vi "Service.EnumToGUID.vi"(11 "Type":T1) -> (3 "GUID":string)   [LabVIEW 2019, in "Diagnostics Addon System Explorer.lvlib"]
uses:
  Diagnostics Addon System Explorer.lvlib
  Addon Shared/SubVIs/Constants.vi
  Addon Shared/Diagnostics Addon Shared.lvlib
  Addon Shared/Types/Type.ctl
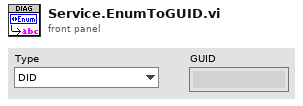
[diagram p1: front panel]
types:
  T1 = typedef "Diagnostics Addon Shared.lvlib/Type.ctl" = enum16{"DID", "CDID", "PID", "CPID", "Read Memory", "Write Memory", "IO Control", "Routine Start", "Routine Request", "Routine Stop", "User Defined", "DTC Control", "Clear DTCs", "Read DTCs", "Start DTCs", "DTC Change Count", "Tester Present", "Unlock ECU", "Reset ECU", "Diag Session Control", "Communication Control", "DPID Control", "Poll Control", "Diag Comm Port Control"}
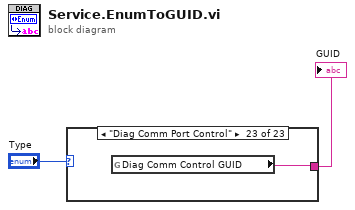
[diagram p0: block diagram]
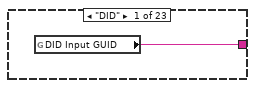
[diagram p2: hidden frame]
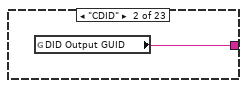
[diagram p3: hidden frame]
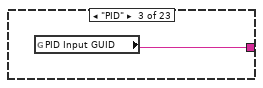
[diagram p4: hidden frame]
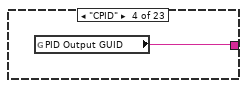
[diagram p5: hidden frame]
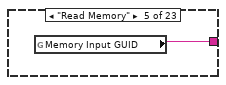
[diagram p6: hidden frame]
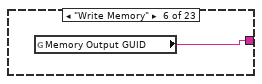
[diagram p7: hidden frame]
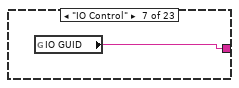
[diagram p8: hidden frame]
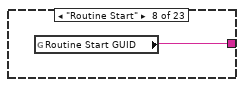
[diagram p9: hidden frame]
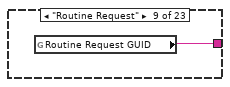
[diagram p10: hidden frame]
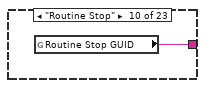
[diagram p11: hidden frame]
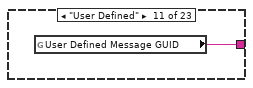
[diagram p12: hidden frame]
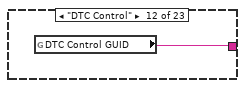
[diagram p13: hidden frame]
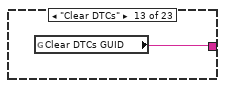
[diagram p14: hidden frame]
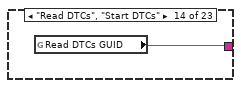
[diagram p15: hidden frame]
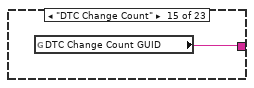
[diagram p16: hidden frame]
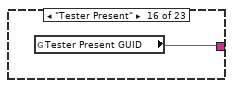
[diagram p17: hidden frame]
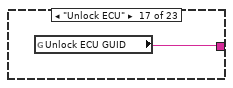
[diagram p18: hidden frame]
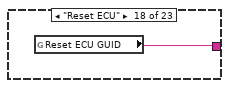
[diagram p19: hidden frame]
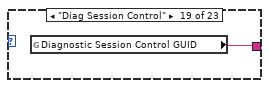
[diagram p20: hidden frame]
diagram:
  n1 = case shown="\"Diag Comm Port Control\"" "Type" {
    tunnel: [w3 w4 w5 w6 w7 w8 w9 w10 w11 w12 w13 w14 w15 w16 w17 w18 w19 w20 w21 w22 w23 w24 w25] -> w1
    frame "DID" {
      n2 = global read "Constants.vi" "DID Input GUID"() -> (w3:string)
    }
    frame "CDID" {
      n3 = global read "Constants.vi" "DID Output GUID"() -> (w4:string)
    }
    frame "PID" {
      n4 = global read "Constants.vi" "PID Input GUID"() -> (w5:string)
    }
    frame "CPID" {
      n5 = global read "Constants.vi" "PID Output GUID"() -> (w6:string)
    }
    frame "Read Memory" {
      n6 = global read "Constants.vi" "Memory Input GUID"() -> (w7:string)
    }
    frame "Write Memory" {
      n7 = global read "Constants.vi" "Memory Output GUID"() -> (w8:string)
    }
    frame "IO Control" {
      n8 = global read "Constants.vi" "IO GUID"() -> (w9:string)
    }
    frame "Routine Start" {
      n9 = global read "Constants.vi" "Routine Start GUID"() -> (w10:string)
    }
    frame "Routine Request" {
      n10 = global read "Constants.vi" "Routine Request GUID"() -> (w11:string)
    }
    frame "Routine Stop" {
      n11 = global read "Constants.vi" "Routine Stop GUID"() -> (w12:string)
    }
    frame "User Defined" {
      n12 = global read "Constants.vi" "User Defined Message GUID"() -> (w13:string)
    }
    frame "DTC Control" {
      n13 = global read "Constants.vi" "DTC Control GUID"() -> (w14:string)
    }
    frame "Clear DTCs" {
      n14 = global read "Constants.vi" "Clear DTCs GUID"() -> (w15:string)
    }
    frame "Read DTCs", "Start DTCs" {
      n15 = global read "Constants.vi" "Read DTCs GUID"() -> (w16:string)
    }
    frame "DTC Change Count" {
      n16 = global read "Constants.vi" "DTC Change Count GUID"() -> (w17:string)
    }
    frame "Tester Present" {
      n17 = global read "Constants.vi" "Tester Present GUID"() -> (w18:string)
    }
    frame "Unlock ECU" {
      n18 = global read "Constants.vi" "Unlock ECU GUID"() -> (w19:string)
    }
    frame "Reset ECU" {
      n19 = global read "Constants.vi" "Reset ECU GUID"() -> (w20:string)
    }
    frame "Diag Session Control" {
      n20 = global read "Constants.vi" "Diagnostic Session Control GUID"() -> (w21:string)
    }
    frame "Communication Control" {
      n21 = global read "Constants.vi" "Normal Communication Control GUID"() -> (w22:string)
    }
    frame "DPID Control" {
      n22 = global read "Constants.vi" "DPID GUID"() -> (w23:string)
    }
    frame "Poll Control" {
      n23 = global read "Constants.vi" "Poll GUID"() -> (w24:string)
    }
    frame "Diag Comm Port Control" {
      n24 = global read "Constants.vi" "Diag Comm Control GUID"() -> (w25:string)
    }
  }
  "GUID" <- w1
